vi "Read Parallel Operation Period(ms).vi"(8 "error in (no error)":errorcluster, 11 "Parallel Operation Actor in":refnum<class "Parallel Operation Actor.lvclass">) -> (0 "error out":errorcluster, 2 "Parallel Operation Period(ms)":i32=100, 3 "Parallel Operation Actor out":refnum<class "Parallel Operation Actor.lvclass">)   [LabVIEW 2024, in "Parallel Operation Actor.lvclass"]
uses:
  Parallel Operation Actor.lvclass
  Parallel Operation Actor.lvclass/Parallel Operation Actor.ctl
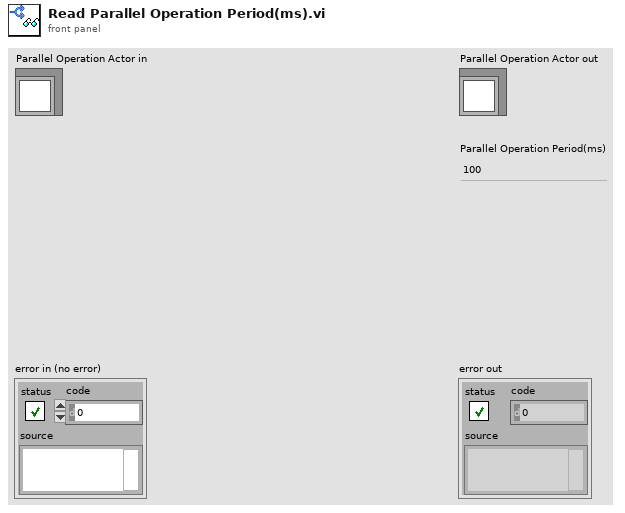
[diagram p1: front panel]
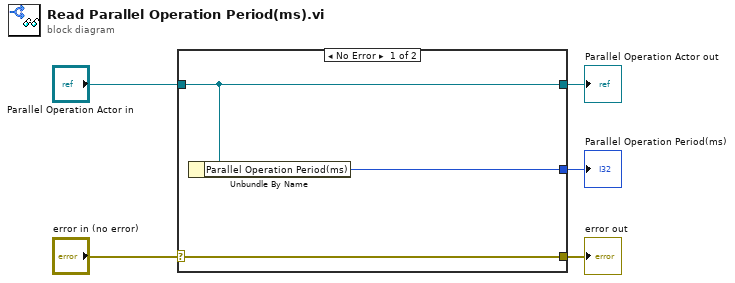
[diagram p0: block diagram]
diagram:
  n1 = case shown="No Error" "error in (no error)" {
    selector: "error in (no error)" -> [w8 w9]
    tunnel: [w8 w9] -> w4
    tunnel: [w7 w10] -> w2
    tunnel: "Parallel Operation Actor in" -> [w7 w10]
    tunnel: [w6 _] -> w1
    frame No Error {
      n2 = Unbundle By Name(w7) -> ("Parallel Operation Period(ms)"=w6:i32)
    }
    frame Error {
    }
  }
  "error out" <- w4
  "Parallel Operation Actor out" <- w2
  "Parallel Operation Period(ms)" <- w1
